vi "_emi_SMLoop Register new.vi"(5 "Loop ID":u16, 9 "error in (no error)":errorcluster) -> (6 "Loop ID Out":u16, 10 "error out":errorcluster)   [LabVIEW 2011]
doc: "Register a new SMLoop. Only real use in QMS Creator.\n\nChecks if loops exists, if it does, does nothing.\n\nTODO: Is that right? Should tit through error? .... Dropped becuase the linking routine needs to be able to created loops, in case it runs befor loop"
uses:
  Loop control/Private/_emi_Loop control int action.ctl
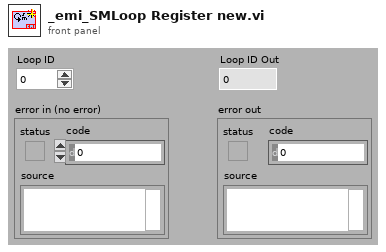
[diagram p1: front panel]
types:
  T1 = typedef "_emi_Loop control int action.ctl" = enum16{"Init index", "Get index", "Set index", "Get Size"}
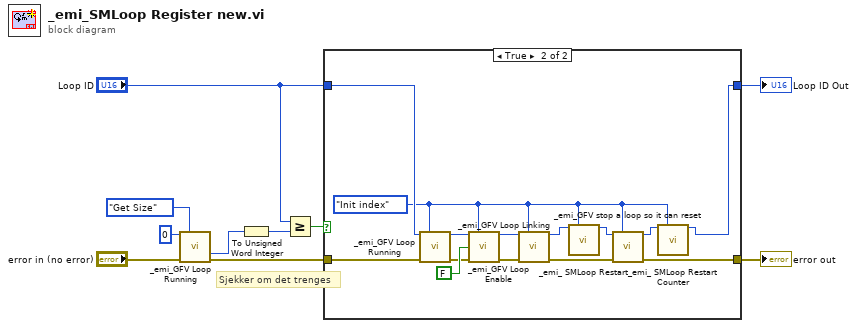
[diagram p0: block diagram]
diagram:
  # "Sjekker om det trenges"
  n1 = call "_emi_GFV Loop Running.vi"("Loop Index/Numb"=u16 0, "Action(Get Index)"=_emi_Loop_control_int_action."Get Size", "error in (no error)"="error in (no error)") -> ("Size"=w4:i32, "error out"=w7:errorcluster)  [unwired: 9 in, 2 out]
  n2 = To Unsigned Word Integer(number=w4) -> (unsigned 16bit integer=w1:u16)
  n3 = Greater Or Equal?(x="Loop ID", y=w1) -> (x >= y?=w2:bool)
  n4 = case shown="True" w2 {
    tunnel: [w11 w14] -> w10
    tunnel: [w12 w15] -> w9
    tunnel: w7 -> [w12 w18]
    tunnel: "Loop ID" -> [w11 w17]
    frame False {
    }
    frame True {
      w13 = _emi_Loop_control_int_action."Init index" ("Action(Get Index)")
      n5 = call "_emi_GFV Loop Running.vi"("Loop Index/Numb"=w17, "Action(Get Index)"=w13, "error in (no error)"=w18) -> ("Index out"=w19:u16, "error out"=w20:errorcluster)  [unwired: 9 in, 2 out]
      n6 = call "_emi_GFV Loop Enable.vi"("Loop Index/Numb"=w19, "Action(Get Index)"=w13, "Loop enable In(T)"=FALSE, "error in (no error)"=w20) -> ("Index out"=w23:u16, "error out"=w22:errorcluster)  [unwired: 8 in, 2 out]
      n7 = call "_emi_GFV Loop Linking.vi"("Loop Index/Numb"=w23, "Action(Get Index)"=w13, "error in (no error)"=w22) -> ("Index out"=w24:u16, "error out"=w25:errorcluster)  [unwired: 9 in, 2 out]
      n8 = call "_emi_ SMLoop Restart.vi"("Loop Index/Numb"=w24, "Action(Get Index)"=w13) -> ("Index out"=w26:u16)  [unwired: 11 in, 2 out]
      n9 = call "_emi_GFV stop a loop so it can reset.vi"("Loop Index/Numb"=w26, "Action(Get Index)"=w13, "error in (no error)"=w25) -> ("Index out"=w16:u16, "error out"=w15:errorcluster)  [unwired: 9 in, 2 out]
      n10 = call "_emi_ SMLoop Restart Counter.vi"("Loop Index/Numb"=w16, "Action(Get Index)"=w13) -> ("Index out"=w14:u16)  [unwired: 11 in, 2 out]
    }
  }
  "Loop ID Out" <- w10
  "error out" <- w9
